vi "Main - On Load.vi"(8 "error in (no error)":errorcluster, 11 "Device Item Ref in":T1 format="%.0x") -> (0 "error out":errorcluster, 3 "Device Item Ref out":T1 format="%.0x")   [LabVIEW 2016, in "Scan Engine Custom Device.lvlib"]
uses:
  Scan Engine Custom Device.lvlib
  <vilib>/NI Veristand/Custom Device API/Custom Device API.lvlib
  <vilib>/NI Veristand/Custom Device API/Custom Device Channel Type.ctl
  <vilib>/NI Veristand/Custom Device API/Custom Device Channel.ctl
  <vilib>/NI Veristand/Custom Device Tools/Custom Device Utility Library/Custom Device Utility Library.lvlib
  Globals/Scan Engine GUIDs.vi
  Globals/Property Strings.vi
  <vilib>/NI Veristand/Custom Device Tools/Custom Device Utility Library/NI VeriStand - Search for All Items by GUID.vi
  <vilib>/NI Veristand/Custom Device API/Get Item Property (U32).vi
  Globals/String Constants.vi
  <vilib>/regexp/Match Regular Expression.xnode
  NationalInstruments.VeriStand.SystemDefinitionAPI
  <vilib>/NI Veristand/Custom Device API/Set Item Property (Boolean).vi
  <vilib>/NI Veristand/Custom Device API/Custom Device Item Ref.ctl
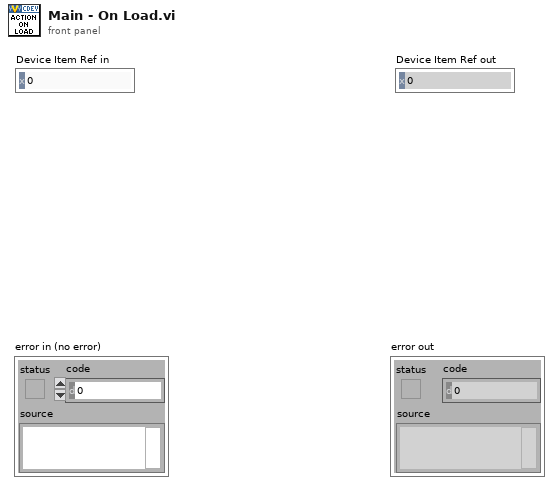
[diagram p1: front panel]
types:
  T1 = typedef "Custom Device API.lvlib/Custom Device Item Ref.ctl" = u64
  T2 = typedef "Custom Device API.lvlib/Custom Device Channel.ctl" = cluster{"Type":T3, "Units":string, "Default Value":dbl, "Faultable":bool, "Scalable":bool}
  T3 = typedef "Custom Device API.lvlib/Custom Device Channel Type.ctl" = enum16{"Input", "Output"}
  T4 = typedef "Modules.lvlibp/Custom Device API.lvlib/Custom Device Item Ref.ctl" = u64
  T5 = typedef "Custom Device API.lvlib/Custom Device Item Info.ctl" = cluster{"Name":string, "Is Channel":bool, "GUID":string, "Is Waveform":bool}
  T6 = typedef "Modules.lvlibp/RSI Module.lvclass/Module Models.ctl" = enum16{"Empty", "NI 9201", "NI 9203", "NI 9205", "NI 9206", "NI 9207", "NI 9208", "NI 9211", "NI 9213", "NI 9214", "NI 9215", "NI 9217", "NI 9219", "NI 9221", "NI 9225", "NI 9227", "NI 9229", "NI 9233", "NI 9234", "NI 9235", "NI 9236", "NI 9237", "NI 9239", "NI 9263", "NI 9264", "NI 9265", "NI 9269", "NI 9375", "NI 9401", "NI 9402", "NI 9403", "NI 9411", "NI 9421", "NI 9422", "NI 9423", "NI 9425", "NI 9426", "NI 9435", "NI 9472", "NI 9474", "NI 9475", "NI 9476", "NI 9477", "NI 9478", "NI 9481", "NI 9482", "NI 9485"}
  T7 = typedef "Modules.lvlibp/RSI Module.lvclass/Slot Settings.ctl" = cluster{"Slot":u32, "EtherCAT?":bool}
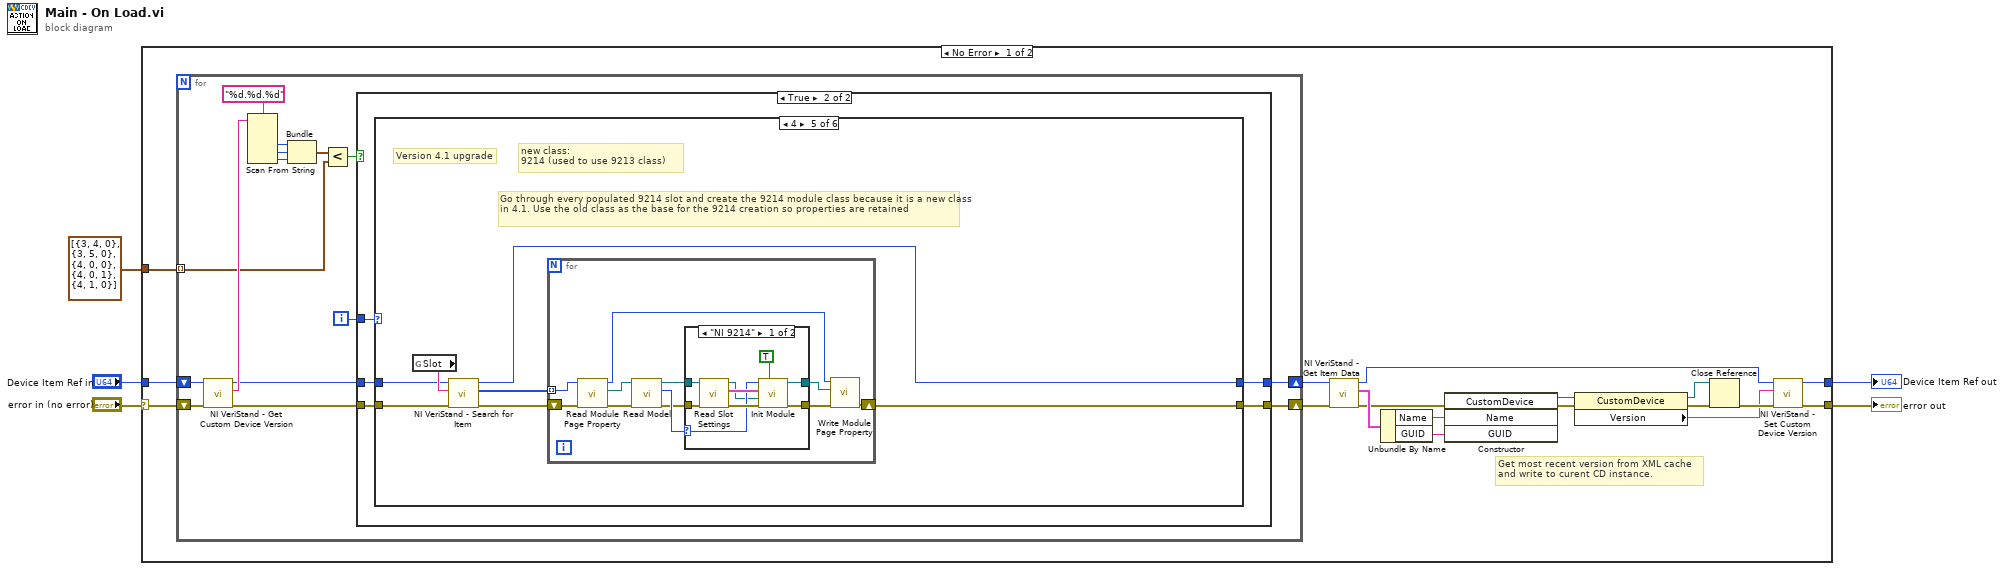
[diagram p0: block diagram]
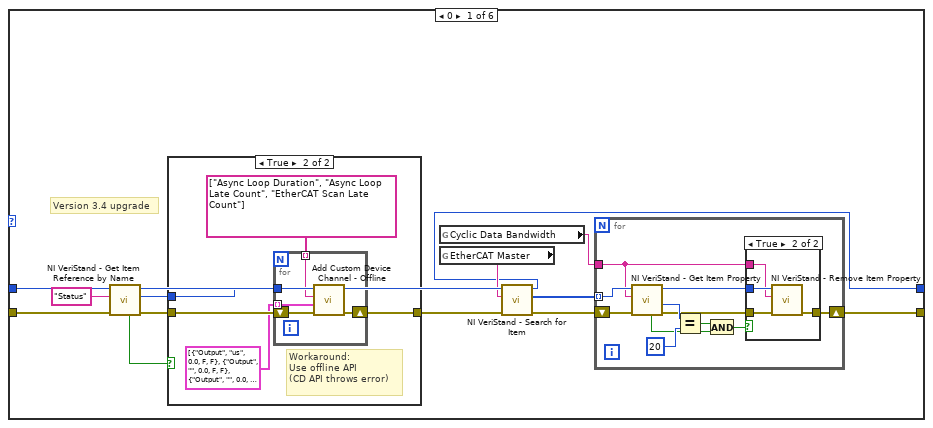
[diagram p3: hidden frame]
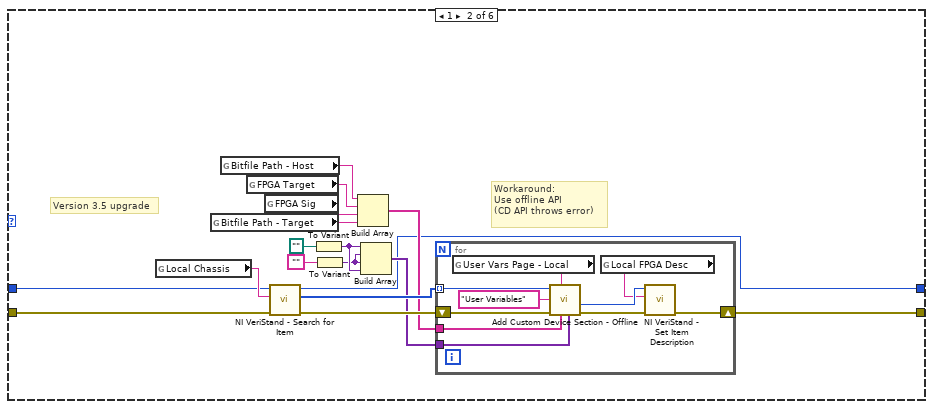
[diagram p6: hidden frame]
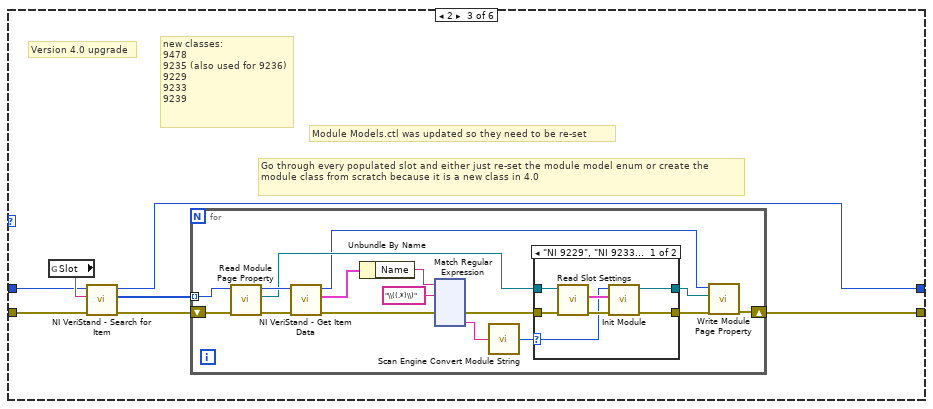
[diagram p7: hidden frame]
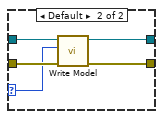
[diagram p8: hidden frame]
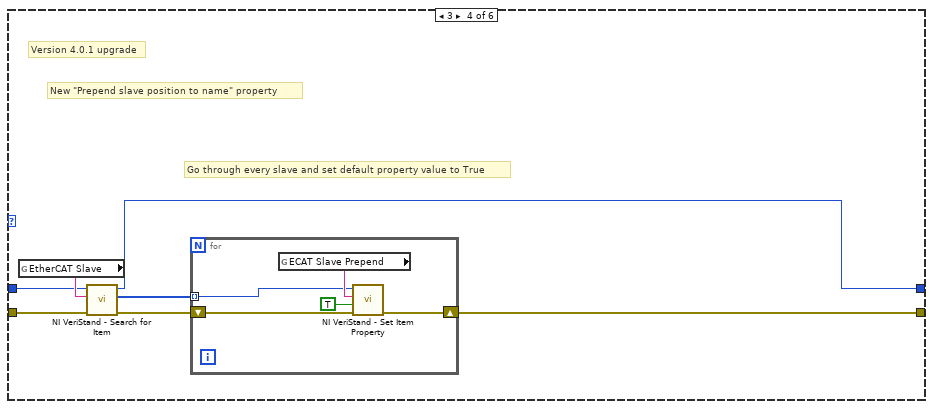
[diagram p9: hidden frame]
diagram:
  n1 = case shown="No Error" "error in (no error)" {
    selector: "error in (no error)" -> [w23 w306]
    tunnel: [w6 w306] -> w3
    tunnel: "Device Item Ref in" -> [w22 w305]
    tunnel: [w7 w305] -> w2
    tunnel: cluster{i32, i32, i32}[] [{3, 4, 0}, {3, 5, 0}, {4, 0, 0}, {4, 0, 1}, {4, 1, 0}] -> [w21 _]
    frame No Error {
      # "Get most recent version from XML cache\nand write to curent CD instance."
      n2 = for {
        shift-right: [w29] -> w19
        shift-left: w23 -> [w34]
        shift-right: [w27] -> w20
        shift-left: w22 -> [w33]
        tunnel: w21 -> [w24] mode=indexing
        i -> [w26]
        n3 = call <vilib>:"NI VeriStand - Get Custom Device Version.vi"("error in (no error)"=w34, "Device Ref in"=w33) -> ("error out"=w30:errorcluster, "Value"=w32:string, "Device Ref out"=w28:T1)  [unwired: 7 in]
        n4 = Scan From String(format string="%d.%d.%d", input string=w32) -> (output 1=w36:i32, output 2=w37:i32, output 3=w25:i32)  [unwired: 5 in, 3 out]
        n5 = Bundle(w36, w37, w25) -> (w38:cluster{i32, i32, i32})  [unwired: 1 in]
        n6 = Less?(x=w38, y=w24) -> (x < y?=w31:bool)
        n7 = case shown="True" w31 {
          tunnel: w30 -> [w40 w45]
          tunnel: [w40 w44] -> w29
          tunnel: w28 -> [w39 w41]
          tunnel: [w39 w42] -> w27
          tunnel: w26 -> [_ w43]
          frame False {
          }
          frame True {
            n8 = case shown="4" w43 {
              tunnel: w45 -> [w46 w89 w116 w264 w276 w304]
              tunnel: [w52 w88 w115 w263 w275 w304] -> w44
              tunnel: [w54 w87 w114 w262 w274 w303] -> w42
              tunnel: w41 -> [w47 w90 w117 w265 w277 w303]
              frame 0 {
                # "Version 3.4 upgrade"
                n9 = call <vilib>:"NI VeriStand - Get Item Reference by Name.vi"("error in (no error)"=w46, "Item Name"="Status" ("Section Name"), "Parent Ref in"=w47) -> ("error out"=w50:errorcluster, "Item Ref"=w49:T1, "Parent Ref out"=w58:T1, "Found"=w48:bool)  [unwired: 5 in]
                n10 = case shown="True" w48 {
                  tunnel: w49 -> [_ w65]
                  tunnel: w50 -> [w60 w64]
                  tunnel: [w60 w63] -> w59
                  frame False {
                  }
                  frame True {
                    # "Workaround:\nUse offline API\n(CD API throws error)"
                    n11 = for {
                      tunnel: w65 -> [w68]
                      shift-right: [w70] -> w63
                      shift-left: w64 -> [w69]
                      tunnel: T2[] [{"Type"=enum."Output", "Units"="us", "Default Value"=0.0, "Faultable"=FALSE, "Scalable"=FALSE}, {"Type"=enum."Output", "Units"="", "Default Value"=0.0, "Faultable"=FALSE, "Scalable"=FALSE}, {"Type"=enum."Output", "Units"="", "Default Value"=0.0, "Faultable"=FALSE, "Scalable"=FALSE}] -> [w66] mode=indexing
                      tunnel: string[] ["Async Loop Duration", "Async Loop Late Count", "EtherCAT Scan Late Count"] -> [w67] mode=indexing
                      n12 = call "Add Custom Device Channel - Offline.vi"("error in (no error)"=w69, "Channel"=w66, "Channel Name"=w67, "Parent Ref in"=w68) -> ("error out"=w70:errorcluster)  [unwired: 4 in, 3 out]
                    }
                  }
                }
                n13 = global read "Property Strings.vi" "Cyclic Data Bandwidth"() -> (w53:string)
                n14 = global read "Scan Engine GUIDs.vi" "EtherCAT Master"() -> (w57:string)
                n15 = call-poly <vilib>:"NI VeriStand - Search for Item.vi"("error in"=w59, "Item GUID"=w57, "Section Ref in"=w58) -> ("error out"=w55:errorcluster, "Item Refs"=w56:T1[], "Section Ref out"=w54:T1)  [unwired: 5 in, 1 out]
                n16 = for {
                  tunnel: w56 -> [w80] mode=indexing
                  shift-right: [w71] -> w52
                  shift-left: w55 -> [w81]
                  tunnel: w53 -> [w72]
                  n17 = call-poly <vilib>:"NI VeriStand - Get Item Property.vi"("error in (no error)"=w81, "Property Name"=w72, "Item Ref in"=w80) -> ("error out"=w74:errorcluster, "Value"=w79:u32, "Item Ref out"=w73:T1, "Found?"=w76:bool)  [unwired: 5 in]
                  n18 = Equal?(x=w79, y=u32 20 ("x")) -> (x = y?=w77:bool)
                  n19 = And(x=w77, y=w76) -> (x .and. y?=w75:bool)
                  n20 = case shown="True" w75 {
                    tunnel: w74 -> [w82 w85]
                    tunnel: w73 -> [_ w86]
                    tunnel: w72 -> [_ w84]
                    tunnel: [w82 w83] -> w71
                    frame False {
                    }
                    frame True {
                      n21 = call <vilib>:"NI VeriStand - Remove Item Property.vi"("error in (no error)"=w85, "Property Name"=w84, "Item Ref in"=w86) -> ("error out"=w83:errorcluster)  [unwired: 6 in, 2 out]
                    }
                  }
                }
              }
              frame 1 {
                # "Workaround:\nUse offline API\n(CD API throws error)"
                # "Version 3.5 upgrade"
                n22 = global read "Scan Engine GUIDs.vi" "Local Chassis"() -> (w101:string)
                n23 = global read "Property Strings.vi" "Bitfile Path - Target"() -> (w94:string)
                n24 = global read "Property Strings.vi" "Bitfile Path - Host"() -> (w97:string)
                n25 = global read "Property Strings.vi" "FPGA Target"() -> (w96:string)
                n26 = global read "Property Strings.vi" "FPGA Sig"() -> (w95:string)
                n27 = call-poly <vilib>:"NI VeriStand - Search for Item.vi"("error in"=w89, "Item GUID"=w101, "Section Ref in"=w90) -> ("error out"=w103:errorcluster, "Item Refs"=w102:T1[], "Section Ref out"=w87:T1)  [unwired: 5 in, 1 out]
                n28 = To Variant(anything=path "") -> (Variant=w93:variant)
                n29 = To Variant(anything="") -> (Variant=w91:variant)
                n30 = Build Array(w97, w96, w95, w94) -> (w99:string[])
                n31 = Build Array(w93, w91, w91, w93) -> (w100:variant[])
                n32 = for {
                  tunnel: w99 -> [w112]
                  tunnel: w100 -> [w111]
                  shift-right: [w106] -> w88
                  shift-left: w103 -> [w113]
                  tunnel: w102 -> [w110] mode=indexing
                  n33 = global read "Scan Engine GUIDs.vi" "User Vars Page - Local"() -> (w109:string)
                  n34 = call "Add Custom Device Section - Offline.vi"("Property Values"=w111, "Property names"=w112, "GUID (Default Section)"=w109, "error in (no error)"=w113, "Section Name"="User Variables", "Parent Ref in"=w110) -> ("error out"=w107:errorcluster, "Section Ptr"=w105:T1)  [unwired: 2 in, 2 out]
                  n35 = global read "String Constants.vi" "Local FPGA Desc"() -> (w104:string)
                  n36 = call <vilib>:"NI VeriStand - Set Item Description.vi"("error in (no error)"=w107, "Description"=w104, "Item Ref in"=w105) -> ("error out"=w106:errorcluster)  [unwired: 6 in, 2 out]
                }
              }
              frame 2 {
                # "new classes:\n9478\n9235 (also used for 9236)\n9229\n9233\n9239"
                # "Go through every populated slot and either just re-set the module model enum or create the module class from scratch because it is a new class in 4.0"
                # "Module Models.ctl was updated so they need to be re-set"
                # "Version 4.0 upgrade"
                n37 = global read "Scan Engine GUIDs.vi" "Slot"() -> (w118:string)
                n38 = call-poly <vilib>:"NI VeriStand - Search for Item.vi"("error in"=w116, "Item GUID"=w118, "Section Ref in"=w117) -> ("error out"=w120:errorcluster, "Item Refs"=w119:T1[], "Section Ref out"=w114:T1)  [unwired: 5 in, 1 out]
                n39 = for {
                  shift-right: [w136] -> w115
                  shift-left: w120 -> [w128]
                  tunnel: w119 -> [w129] mode=indexing
                  n40 = call "Read Module Page Property.vi"("error in (no error)"=w128, "Node Ptr In"=w129) -> ("error out"=w131:errorcluster, "RSI Module"=w123:refnum<class "RSI Module.lvclass">, "Node Ptr Out"=w130:T4)  [unwired: 7 in]
                  n41 = call <vilib>:"NI VeriStand - Get Item Data.vi"("error in (no error)"=w131, "Item Ref in"=w130) -> ("error out"=w134:errorcluster, "Item Info"=w135:T5, "Item Ref out"=w121:T1)  [unwired: 6 in, 1 out]
                  n42 = Unbundle By Name(w135) -> ("Name"=w133:string)
                  n43 = xnode "Match Regular Expression"("input string"=w133, "regular expression"="\\((.*)\\)", "error in"=w134) -> ("error out"=w127:errorcluster, "submatch 1"=w126:string)  [unwired: 3 in, 4 out]
                  n44 = call "Scan Engine Convert Module String.vi"("Module Name"=w126) -> ("Module"=w125:T6)
                  n45 = case shown="\"NI 9229\", \"NI 9233\", \"NI 9235\", \"NI 9236\", \"NI 9239\", \"NI 9478\"" w125 {
                    selector: w125 -> [w139 w146]
                    tunnel: w127 -> [w141 w148]
                    tunnel: [w138 w147] -> w124
                    tunnel: w123 -> [w140 w145]
                    tunnel: [w137 w144] -> w122
                    frame "NI 9229", "NI 9233", "NI 9235", "NI 9236", "NI 9239", "NI 9478" {
                      n46 = call "Read Slot Settings.vi"("error in (no error)"=w141, "RSI Module in"=w140) -> ("error out"=w142:errorcluster, "Slot Settings"=w143:T7)  [unwired: 7 in, 1 out]
                      n47 = call "Init Module.vi"("error in (no error)"=w142, "Slot Settings"=w143, "Module Model"=w139) -> ("error out"=w138:errorcluster, "RSI Module out"=w137:refnum<class "RSI Module.lvclass">)  [unwired: 7 in]
                    }
                    frame Default {
                      n48 = call "Write Model.vi"("error in (no error)"=w148, "Model"=w146, "RSI Module in"=w145) -> ("error out"=w147:errorcluster, "RSI Module out"=w144:refnum<class "RSI Module.lvclass">)  [unwired: 7 in]
                    }
                  }
                  n49 = call "Write Module Page Property.vi"("error in (no error)"=w124, "RSI Module"=w122, "Node Ptr In"=w121) -> ("error out"=w136:errorcluster)  [unwired: 6 in, 2 out]
                }
              }
              frame 3 {
                # "New \"Prepend slave position to name\" property"
                # "Go through every slave and set default property value to True"
                # "Version 4.0.1 upgrade"
                n50 = global read "Scan Engine GUIDs.vi" "EtherCAT Slave"() -> (w266:string)
                n51 = call-poly <vilib>:"NI VeriStand - Search for Item.vi"("error in"=w264, "Item GUID"=w266, "Section Ref in"=w265) -> ("error out"=w268:errorcluster, "Item Refs"=w267:T1[], "Section Ref out"=w262:T1)  [unwired: 5 in, 1 out]
                n52 = for {
                  shift-right: [w269] -> w263
                  shift-left: w268 -> [w273]
                  tunnel: w267 -> [w271] mode=indexing
                  n53 = global read "Property Strings.vi" "ECAT Slave Prepend"() -> (w272:string)
                  n54 = call-poly <vilib>:"NI VeriStand - Set Item Property.vi"("error in (no error)"=w273, "Value"=TRUE, "Property Name"=w272, "Item Ref in"=w271) -> ("error out"=w269:errorcluster)  [unwired: 5 in, 2 out]
                }
              }
              frame 4 {
                # "new class:\n9214 (used to use 9213 class)"
                # "Go through every populated 9214 slot and create the 9214 module class because it is a new class in 4.1. Use the old class as the base for the 9214 creation so properties are retained"
                # "Version 4.1 upgrade"
                n55 = global read "Scan Engine GUIDs.vi" "Slot"() -> (w278:string)
                n56 = call-poly <vilib>:"NI VeriStand - Search for Item.vi"("error in"=w276, "Item GUID"=w278, "Section Ref in"=w277) -> ("error out"=w280:errorcluster, "Item Refs"=w279:T1[], "Section Ref out"=w274:T1)  [unwired: 5 in, 1 out]
                n57 = for {
                  shift-right: [w291] -> w275
                  shift-left: w280 -> [w289]
                  tunnel: w279 -> [w290] mode=indexing
                  n58 = call "Read Module Page Property.vi"("error in (no error)"=w289, "Node Ptr In"=w290) -> ("error out"=w286:errorcluster, "RSI Module"=w285:refnum<class "RSI Module.lvclass">, "Node Ptr Out"=w281:T4)  [unwired: 7 in]
                  n59 = call "Read Model.vi"("error in (no error)"=w286, "RSI Module in"=w285) -> ("error out"=w282:errorcluster, "Model"=w283:T6, "RSI Module out"=w284:refnum<class "RSI Module.lvclass">)  [unwired: 7 in]
                  n60 = case shown="\"NI 9214\"" w283 {
                    selector: w283 -> [w298 _]
                    tunnel: w282 -> [w297 w302]
                    tunnel: [w293 w302] -> w288
                    tunnel: w284 -> [w294 w301]
                    tunnel: [w292 w301] -> w287
                    frame "NI 9214" {
                      n61 = call "Read Slot Settings.vi"("error in (no error)"=w297, "RSI Module in"=w294) -> ("error out"=w299:errorcluster, "Slot Settings"=w300:T7, "RSI Module out"=w295:refnum<class "RSI Module.lvclass">)  [unwired: 7 in]
                      n62 = call "Init Module.vi"("Create from class input? (F)"=TRUE, "error in (no error)"=w299, "RSI Module in"=w295, "Slot Settings"=w300, "Module Model"=w298) -> ("error out"=w293:errorcluster, "RSI Module out"=w292:refnum<class "RSI Module.lvclass">)  [unwired: 5 in]
                    }
                    frame Default {
                    }
                  }
                  n63 = call "Write Module Page Property.vi"("error in (no error)"=w288, "RSI Module"=w287, "Node Ptr In"=w281) -> ("error out"=w291:errorcluster)  [unwired: 6 in, 2 out]
                }
              }
              frame Default {
              }
            }
          }
        }
      }
      n64 = call <vilib>:"NI VeriStand - Get Item Data.vi"("error in (no error)"=w19, "Item Ref in"=w20) -> ("error out"=w15:errorcluster, "Item Info"=w18:T5, "Item Ref out"=w8:T1)  [unwired: 6 in, 1 out]
      n65 = Unbundle By Name(w18) -> ("Name"=w17:string, "GUID"=w16:string)
      n66 = constructor class="CustomDevice"(error in=w15, "Name"=w17, "GUID"=w16) -> (reference out=w14:refnum<k24>, error out=w13:errorcluster)  [unwired: 2 in, 3 out]
      n67 = property class="CustomDevice"(reference=w14, error in=w13) -> (reference out=w11:refnum<k24>, error out=w12:errorcluster, "Version"=w9:string)
      n68 = Close Reference(reference=w11, error in (no error)=w12) -> (error out=w10:errorcluster)
      n69 = call <vilib>:"NI VeriStand - Set Custom Device Version.vi"("error in (no error)"=w10, "Value"=w9, "Device Ref in"=w8) -> ("error out"=w6:errorcluster, "Device Ref out"=w7:T1)  [unwired: 7 in]
    }
    frame Error {
    }
  }
  "error out" <- w3
  "Device Item Ref out" <- w2
